vi "Climb Handler.vi"(0 "JoystickDevRef":T1={"Device"=enum."USB 1"}) -> ()   [LabVIEW 2019]
uses:
  <vilib>/Rock Robotics/WPI/Joystick/WPI_JoystickDevRef.ctl
  <vilib>/Rock Robotics/WPI/Joystick/WPI_JoystickDeviceEnum.ctl
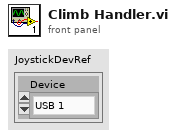
[diagram p1: front panel]
types:
  T1 = typedef "WPI_JoystickDevRef.ctl" = cluster{"Device":T2}
  T2 = typedef "WPI_JoystickDeviceEnum.ctl" = enum16{"USB 0", "USB 1", "USB 2", "USB 3", "USB 4", "USB 5"}
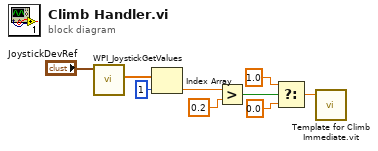
[diagram p0: block diagram]
diagram:
  n1 = call <vilib>:"WPI_JoystickGetValues.vi"("JoystickDevRef"="JoystickDevRef") -> ("Axes"=w8:dbl[])  [unwired: 6 in, 4 out]
  n2 = Index Array(array=w8, index=1) -> (element=w6:dbl)
  n3 = Greater?(x=w6, y=0.2) -> (0:w4:bool)
  n4 = Select(t=1.0, s=w4, f=0.0) -> (s? t:f=w1:dbl)
  n5 = call "Template for Climb Immediate.vit"("Setpoint"=w1) -> ()  [unwired: 10 in, 1 out]
